vi "WebSocket Read Json.vi"(8 "error in":errorcluster, 10 "timeout ms (5000)":i32=5000, 11 "WebSocket Connection in":refnum<k5>) -> (0 "error out":errorcluster, 2 "Websocket Command":T1, 3 "WebSocket Connection out":refnum<k5>)   [LabVIEW 2018]
uses:
  Data Def/Websocket Command.ctl
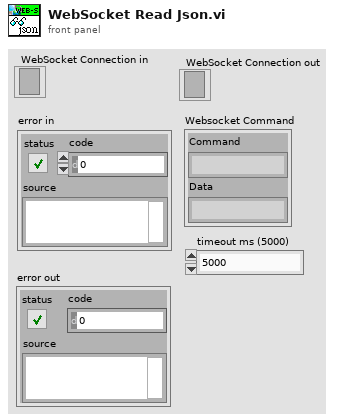
[diagram p1: front panel]
types:
  T1 = typedef "Websocket Command.ctl" = cluster{"Command":string, "Data":string}
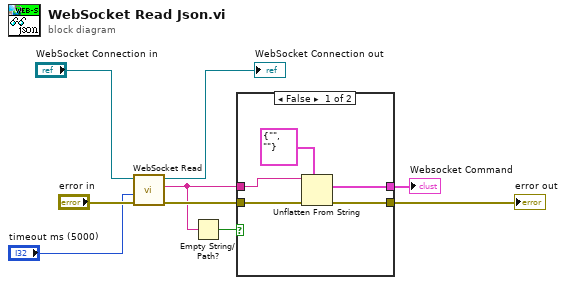
[diagram p0: block diagram]
diagram:
  n1 = call "WebSocket Read.vi"("error in (no error)"="error in", "timeout ms (5000)"="timeout ms (5000)", "WebSocket Connection in"="WebSocket Connection in") -> ("error out"=w7:errorcluster, "Data"=w6:string, "WebSocket Connection out"=→"WebSocket Connection out":refnum<k5>)  [unwired: 5 in, 1 out]
  n2 = Empty String/Path?(string/path=w6) -> (empty?=w8:bool)
  n3 = case shown="False" w8 {
    tunnel: w7 -> [w14 w15]
    tunnel: w6 -> [w13 _]
    tunnel: [w12 w15] -> w4
    tunnel: [w10 _] -> w5
    frame False {
      n4 = Unflatten From String(type=T1 {"Command"="", "Data"=""} ("Websocket Command"), binary string=w13, error in (no error)=w14) -> (value=w10:T1, error out=w12:errorcluster)  [unwired: 2 in, 1 out]
    }
    frame True {
    }
  }
  "Websocket Command" <- w5
  "error out" <- w4
